vi "dxdx2angle.vi"(10 "dy":dbl, 11 "dx":dbl) -> (2 "Angle radians out":dbl, 3 "Angle Degrees out":dbl)   [LabVIEW 2023]
doc: "Calculates the angle (in radians and degrees) of the line defined by dx and dy"
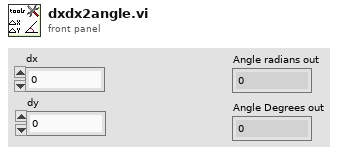
[diagram p1: front panel]
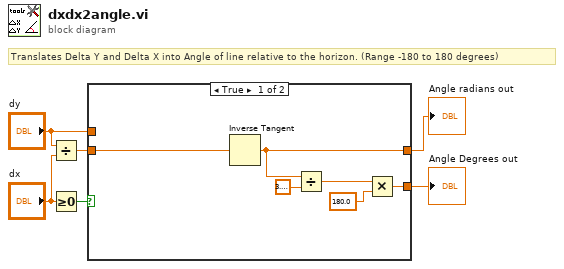
[diagram p0: block diagram]
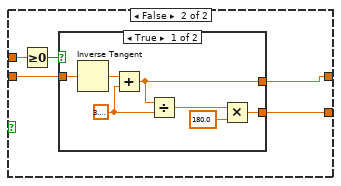
[diagram p2: hidden frame]
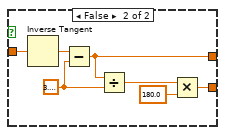
[diagram p3: hidden frame]
diagram:
  # "Translates Delta Y and Delta X into Angle of line relative to the horizon. (Range -180 to 180 degrees)"
  n1 = Divide(x="dy", y="dx") -> (x/y=w4:dbl)
  n2 = Greater Or Equal To 0?(x="dx") -> (x >= 0?=w5:bool)
  n3 = case shown="True" w5 {
    tunnel: w4 -> [w12 w17]
    tunnel: [w8 w16] -> w6
    tunnel: "dy" -> [_ w15]
    tunnel: [w7 w13] -> w3
    frame True {
      n4 = Inverse Tangent(1:w12) -> (0:w7:dbl)
      n5 = Divide(x=w7, y=3.141592653589793 ("Pi")) -> (x/y=w10:dbl)
      n6 = Multiply(x=w10, y=180.0) -> (x*y=w8:dbl)
    }
    frame False {
      n7 = Greater Or Equal To 0?(x=w15) -> (x >= 0?=w14:bool)
      n8 = case shown="True" w14 {
        tunnel: w17 -> [w24 w31]
        tunnel: [w19 w26] -> w16
        tunnel: [w18 w25] -> w13
        frame True {
          w20 = 3.141592653589793 ("Pi")
          n9 = Inverse Tangent(1:w24) -> (0:w21:dbl)
          n10 = Add(x=w21, y=w20) -> (x+y=w18:dbl)
          n11 = Divide(x=w18, y=w20) -> (x/y=w23:dbl)
          n12 = Multiply(x=w23, y=180.0) -> (x*y=w19:dbl)
        }
        frame False {
          w27 = 3.141592653589793 ("Pi")
          n13 = Inverse Tangent(1:w31) -> (0:w29:dbl)
          n14 = Subtract(x=w29, y=w27) -> (x-y=w25:dbl)
          n15 = Divide(x=w25, y=w27) -> (x/y=w30:dbl)
          n16 = Multiply(x=w30, y=180.0) -> (x*y=w26:dbl)
        }
      }
    }
  }
  "Angle Degrees out" <- w6
  "Angle radians out" <- w3
